vi "Launch As Nested.vi"(6 "DataProc Options":T1, 7 "Nested Config Name (DataProc)":string="DataProc", 8 "error in (no error)":errorcluster, 10 "Group":refnum<class "Group DBL.lvclass">, 11 "Parent in":refnum<class "Module.lvclass">) -> (0 "error out":errorcluster, 2 "MessageQ":refnum<class "MessageQ.lvclass">, 3 "Parent out":refnum<class "Module.lvclass">)   [LabVIEW 2020, in "VolatusData.lvlib" / "Data Processor Module.lvclass"]
uses:
  Data Processor Module.lvclass
  Volatus/Module/Module.lvclass
  Volatus/MessageQ/MessageQ.lvclass
  lv-vecto/Vecto/Group DBL/Group DBL.lvclass
  DataProc Options.ctl
  VolatusConfig/Task/Task.lvclass
  C:/dev/lv20CE/relink/lv-volatus/VolatusConfig/VolatusConfigElement/VolatusConfigElement.lvclass
  Volatus/Module/Module.lvclass/Module.ctl
  VolatusConfig/VolatusConfigElement/VolatusConfigElement.lvclass/VolatusConfigElement.ctl
  Volatus/Module/Config.vi
  VolatusConfig/VolatusConfigElement/Element.vi
  C:/dev/lv20CE/relink/lv-volatus/Volatus/Module/Module.lvclass
  VolatusConfig/VolatusConfigElement/VolatusConfigElement.lvclass
  VolatusData.lvlib
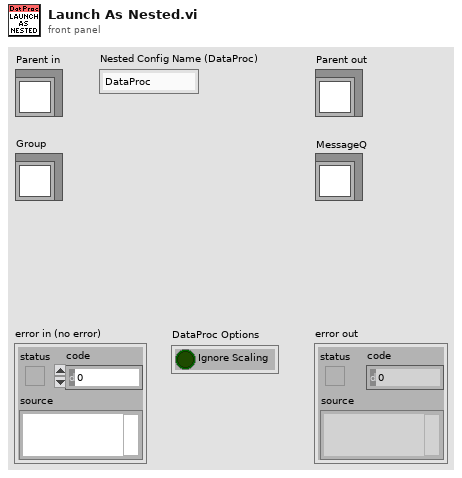
[diagram p1: front panel]
types:
  T1 = typedef "VolatusData.lvlib/DataProc Options.ctl" = cluster{"Ignore Scaling":bool}
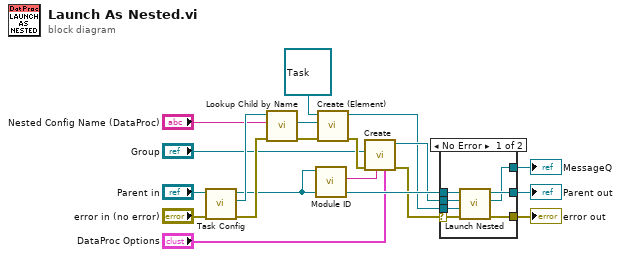
[diagram p0: block diagram]
diagram:
  n1 = call "Task Config.vi"("error in (no error)"="error in (no error)", "Module in"="Parent in") -> ("error out"=w8:errorcluster, "Task Config"=w13:refnum<class "Task.lvclass">, "Module out"=w6:refnum<class "Module.lvclass">)  [unwired: 7 in]
  n2 = call "Lookup Child by Name.vi"("error in (no error)"=w8, "Child Name"="Nested Config Name (DataProc)", "VolatusConfigElement in"=w13) -> ("error out"=w18:errorcluster, "Child"=w16:refnum<class "Config Element.lvclass">)  [unwired: 5 in, 2 out]
  n3 = call-dynamic "Module ID.vi"("Module in"=w6) -> ("Module ID"=w12:string)  [unwired: 10 in]
  n4 = call "Create (Element).vi"("error in (no error)"=w18, "Element"=w16, "VolatusConfigElement in"=refnum<class "Task.lvclass"> refnum ("VolatusConfigElement out")) -> ("error out"=w19:errorcluster, "VolatusConfigElement out"=w4:refnum<class "Task.lvclass">)  [unwired: 7 in]
  n5 = call "Create.vi"("DataProc Options"="DataProc Options", "Parent Name"=w12, "error in (no error)"=w19, "Group"="Group") -> ("error out"=w3:errorcluster, "Data Processor Module out"=w5:refnum<class "Data Processor Module.lvclass">)  [unwired: 6 in]
  n6 = case shown="No Error" w3 {
    selector: w3 -> [w21 w27]
    tunnel: [w26 w27] -> w11
    tunnel: [w25 w28] -> w10
    tunnel: w6 -> [w24 w28]
    tunnel: w5 -> [w23 _]
    tunnel: w4 -> [w22 _]
    tunnel: [w20 _] -> w2
    frame No Error {
      n7 = call "Launch Nested.vi"("error in (no error)"=w21, "Config Element"=w22, "Nested Module"=w23, "Parent in"=w24) -> ("error out"=w26:errorcluster, "MessageQ"=w20:refnum<class "MessageQ.lvclass">, "Parent out"=w25:refnum<class "Module.lvclass">)  [unwired: 5 in]
    }
    frame Error {
    }
  }
  "error out" <- w11
  "Parent out" <- w10
  "MessageQ" <- w2
